vi "Download_Report_subvi.vi"(8 "error in (no error)":errorcluster, 10 "Value":string[][](array[string]), 11 "Column Header Strings[]":string[][](array[string])) -> (0 "error out":errorcluster)   [LabVIEW 2017]
uses:
  <vilib>/Utility/file.llb/Write Delimited Spreadsheet (string).vi
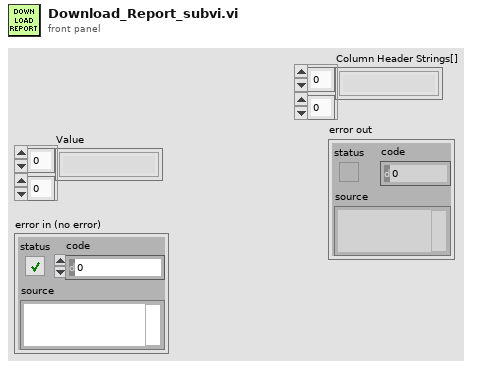
[diagram p1: front panel]
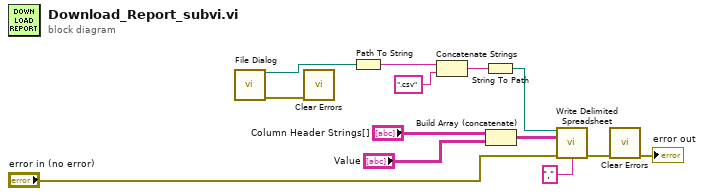
[diagram p0: block diagram]
diagram:
  n1 = call "File Dialog"() -> ("selected path"=w5:path, "error out"=w6:errorcluster)  [unwired: 12 in, 2 out]
  n2 = call <vilib>:"Clear Errors.vi"("error in (no error)"=w6) -> ()  [unwired: 5 in, 2 out]
  n3 = Path To String(path=w5) -> (string=w4:string)
  n4 = Concatenate Strings(w4, ".csv" ("string")) -> (w3:string)
  n5 = String To Path(string=w3) -> (path=w2:path)
  n6 = Build Array (concatenate)("Column Header Strings[]", "Value") -> (w10:string[][])
  n7 = call-poly <vilib>:"Write Delimited Spreadsheet.vi"("file path (dialog if empty)"=w2, "2D data"=w10, "error in (no error)"="error in (no error)", "delimiter (\\t)"="," ("delimiter (\\t)")) -> ("error out"=w13:errorcluster)  [unwired: 10 in, 1 out]
  n8 = call <vilib>:"Clear Errors.vi"("error in (no error)"=w13) -> ("error out"=→"error out":errorcluster)  [unwired: 5 in, 1 out]
